vi "CBC解密.vi"(8 "error in (no error)":errorcluster caption="错误输入（无错误）", 9 "IV":string="78352310323ABCDE", 10 "钥匙":string="78352310323ABCDE", 11 "密文 in":string) -> (0 "error out":errorcluster caption="错误输出", 3 "明文":string)   [LabVIEW 2016, in "数据传输系统-05.lvlib"]
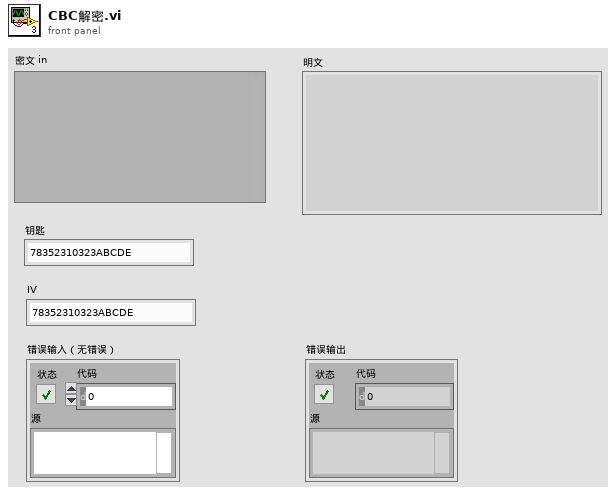
[diagram p1: front panel]
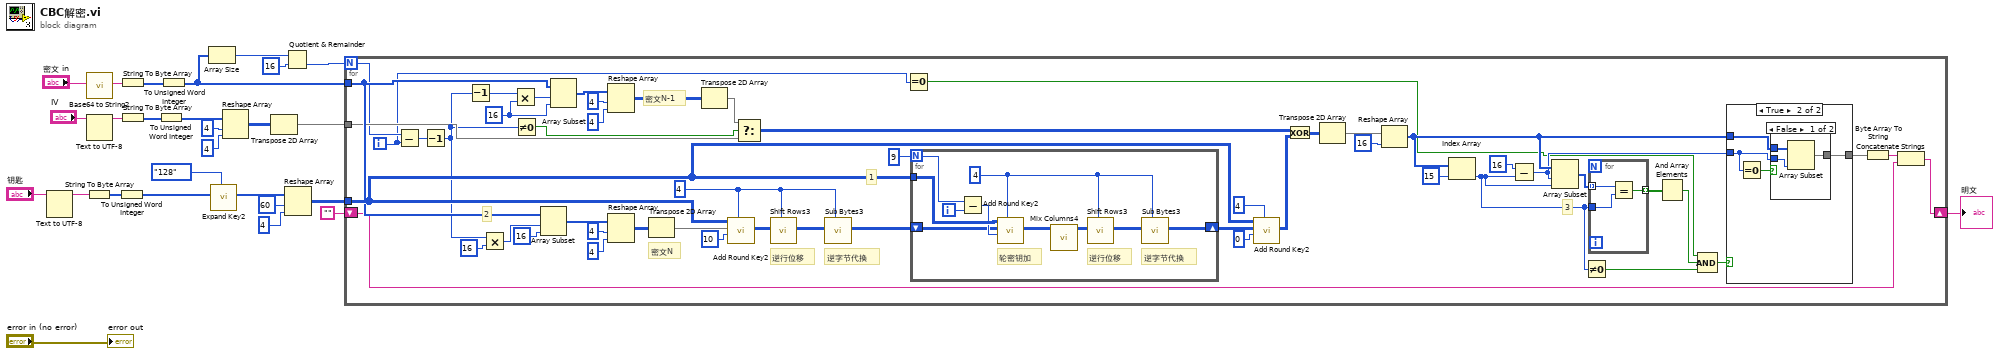
[diagram p0: block diagram]
diagram:
  n1 = Text to UTF-8(11:"钥匙") -> (3:w4:string)  [unwired: 2 in, 1 out]
  n2 = call "Base64 to String2.vi"("Base64 String"="密文 in") -> ("String"=w16:string)  [unwired: 9 in, 1 out]
  n3 = Text to UTF-8(11:"IV") -> (3:w22:string)  [unwired: 2 in, 1 out]
  n4 = String To Byte Array(string=w4) -> (unsigned byte array=w5:u8[])
  n5 = To Unsigned Word Integer(number=w5) -> (unsigned 16bit integer=w3:u16[])
  n6 = String To Byte Array(string=w16) -> (unsigned byte array=w15:u8[])
  n7 = String To Byte Array(string=w22) -> (unsigned byte array=w18:u8[])
  n8 = To Unsigned Word Integer(number=w18) -> (unsigned 16bit integer=w17:u16[])
  n9 = To Unsigned Word Integer(number=w15) -> (unsigned 16bit integer=w9:u16[])
  n10 = Array Size(array=w9) -> (size(s)=w13:i32)
  n11 = call "Expand Key2.vi"("Mode (auto)"=enum16{"128", "192", "256", "auto"}."128", "Key"=w3) -> ("Expanded Key"=w24:u32[])  [unwired: 8 in, 1 out]
  n12 = Reshape Array(w17, 4 ("dimension size"), 4 ("dimension size")) -> (w19:u16[][])
  n13 = Transpose 2D Array(2D array=w19) -> (transposed array=w12:u16[][])
  n14 = Quotient & Remainder(x=w13, y=u16 16) -> (floor(x/y)=w8:i32)  [unwired: 1 out]
  n15 = Reshape Array(w24, 60 ("dimension size"), 4 ("dimension size")) -> (w23:u32[][])
  n16 = for {
    N: w8 -> [w32]
    tunnel: w23 -> [w73]
    tunnel: w9 -> [w64]
    tunnel: w12 -> [w59]
    shift-right: [w53] -> w10
    shift-left: "" -> [w54]
    i -> [w29]
    w41 = 16 ("长度")
    w77 = 4 ("Nb")
    # "密文N"
    # "1"
    # "2"
    # "密文N-1"
    # "3"
    # "逆字节代换"
    # "逆行位移"
    n17 = Subtract(x=w32, y=w29) -> (x-y=w40:i32)
    n18 = Decrement(x=w40) -> (x-1=w36:i32)
    n19 = Decrement(x=w36) -> (x-1=w35:i32)
    n20 = Multiply(x=w36, y=16 ("长度")) -> (x*y=w37:i32)
    n21 = Multiply(x=w35, y=w41) -> (x*y=w39:i32)
    n22 = Not Equal To 0?(x=w36) -> (x != 0?=w60:bool)
    n23 = Array Subset(array=w64, index=w37, length=16 ("长度")) -> (w67:u16[])
    n24 = Array Subset(array=w64, index=w39, length=w41) -> (w61:u16[])
    n25 = Reshape Array(w61, 4 ("dimension size"), 4 ("dimension size")) -> (w45:u16[][])
    n26 = Reshape Array(w67, 4 ("dimension size"), 4 ("dimension size")) -> (w66:u16[][])
    n27 = Transpose 2D Array(2D array=w66) -> (transposed array=w65:u16[][])
    n28 = Transpose 2D Array(2D array=w45) -> (transposed array=w42:u16[][])
    n29 = call "Add Round Key2.vi"("Nb"=w77, "rnd (0)"=10, "State.In"=w65, "ExpandedKey(w)"=w73) -> ("State.Out"=w79:u16[][])  [unwired: 6 in, 1 out]
    n30 = Select(t=w42, s=w60, f=w59) -> (s? t:f=w43:u16[][])
    n31 = call "Shift Rows3.vi"("Nb"=w77, "State In"=w79) -> ("State Out"=w78:u16[][])  [unwired: 8 in, 1 out]
    n32 = call "Sub Bytes3.vi"("Nb"=w77, "State In"=w78) -> ("State Out"=w76:u16[][])  [unwired: 8 in, 1 out]
    n33 = Equal To 0?(x=w29) -> (x = 0?=w28:bool)
    n34 = for {
      N: 9 -> [w97]
      shift-right: [w92] -> w74
      shift-left: w76 -> [w95]
      tunnel: w73 -> [w99]
      i -> [w98]
      w101 = 4 ("Nb")
      # "轮密钥加"
      # "逆字节代换"
      # "逆行位移"
      n35 = Subtract(x=w97, y=w98) -> (x-y=w96:i32)
      n36 = call "Add Round Key2.vi"("Nb"=w101, "rnd (0)"=w96, "State.In"=w95, "ExpandedKey(w)"=w99) -> ("State.Out"=w94:u16[][])  [unwired: 6 in, 1 out]
      n37 = call "Mix Columns4.vi"("State In"=w94) -> ("数组"=w93:u16[][])  [unwired: 10 in]
      n38 = call "Shift Rows3.vi"("Nb"=w101, "State In"=w93) -> ("State Out"=w100:u16[][])  [unwired: 8 in, 1 out]
      n39 = call "Sub Bytes3.vi"("Nb"=w101, "State In"=w100) -> ("State Out"=w92:u16[][])  [unwired: 8 in, 1 out]
    }
    n40 = call "Add Round Key2.vi"("Nb"=4, "rnd (0)"=0, "State.In"=w74, "ExpandedKey(w)"=w73) -> ("State.Out"=w44:u16[][])  [unwired: 6 in, 1 out]
    n41 = Exclusive Or(1:w44, 2:w43) -> (0:w56:u16[][])
    n42 = Transpose 2D Array(2D array=w56) -> (transposed array=w58:u16[][])
    n43 = Reshape Array(w58, 16 ("维数大小")) -> (w48:u16[])
    n44 = Index Array(array=w48, index=15 ("索引")) -> (element=w47:u16)
    n45 = Subtract(x=16, y=w47) -> (x-y=w33:i32)
    n46 = Array Subset(array=w48, index=w33, length=w47) -> (w50:u16[])
    n47 = Not Equal To 0?(x=w47) -> (x != 0?=w30:bool)
    n48 = for {
      tunnel: w47 -> [w91]
      tunnel: w50 -> [w90] mode=indexing
      tunnel: [w89] -> w49 mode=indexing
      n49 = Equal?(x=w90, y=w91) -> (x = y?=w89:bool)
    }
    n50 = And Array Elements(Boolean array=w49) -> (logical AND=w31:bool)
    n51 = Compound Arithmetic op=AND ("复合运算")(w28, w31, w30) -> (w46:bool)
    n52 = case shown="True" w46 {
      tunnel: w48 -> [w81 w85]
      tunnel: w33 -> [_ w83]
      tunnel: [w81 w84] -> w34
      frame False {
      }
      frame True {
        n53 = Equal To 0?(x=w83) -> (x = 0?=w82:bool)
        n54 = case shown="False" w82 {
          tunnel: w85 -> [w88 _]
          tunnel: [w87 _] -> w84
          tunnel: w83 -> [w86 _]
          frame False {
            n55 = Array Subset(array=w88, length=w86) -> (w87:u16[])  [unwired: 1 in]
          }
          frame True {
          }
        }
      }
    }
    n56 = Byte Array To String(unsigned byte array=w34) -> (string=w55:string)
    n57 = Concatenate Strings(w55, w54) -> (w53:string)
  }
  "明文" <- w10
  "error out" <- "error in (no error)"
